vi "Traverse QSM - Nano.vi"(8 "error in":errorcluster, 10 "Nachrichten-Queues (Eingang)":T1) -> (0 "error out":errorcluster)   [LabVIEW 2014]
uses:
  All Message Queues.ctl
  Documents/LabVIEW Data/Unbenanntes Projekt 8/support/Message Queue/Message Cluster.ctl
  Documents/LabVIEW Data/Unbenanntes Projekt 8/support/Message Queue/Enqueue Message (Single).vi
  Documents/LabVIEW Data/Unbenanntes Projekt 8/support/Message Queue/Message Queue.lvlib
panel:
  out "i Blink":i32
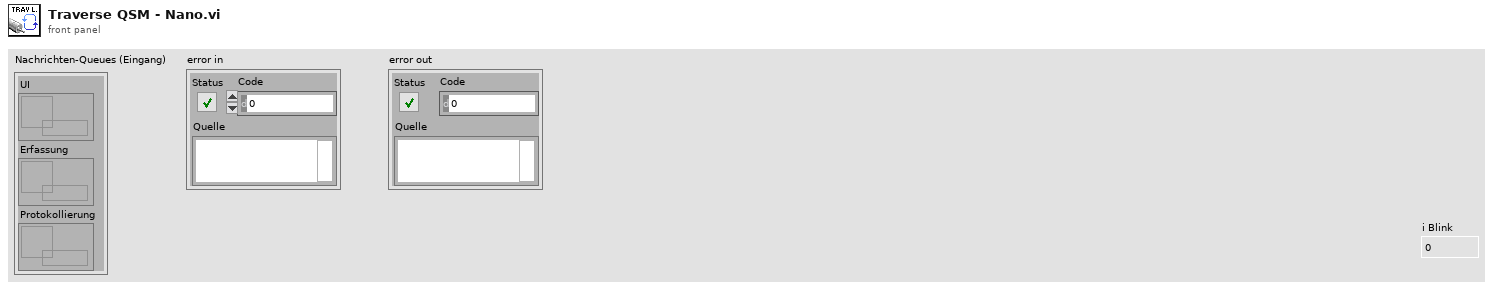
[diagram p1: front panel]
types:
  T1 = typedef "Message Queue.lvlib/All Message Queues.ctl" = cluster{"UI":refnum<queue>, "Erfassung":refnum<queue>, "Traverse":refnum<queue>}
  T2 = cluster{"Status":bool, "Code":i32, "Quelle":string}
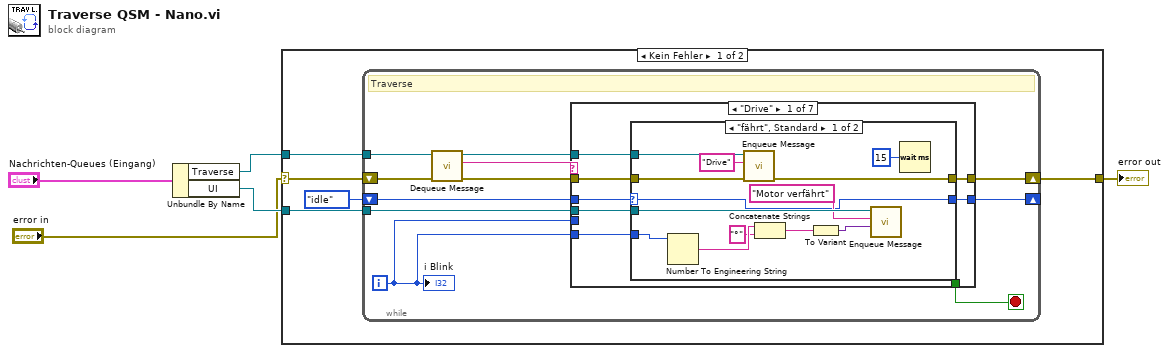
[diagram p0: block diagram]
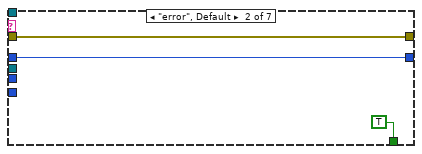
[diagram p3: hidden frame]
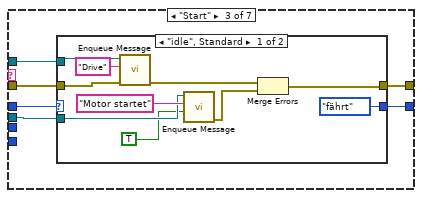
[diagram p4: hidden frame]
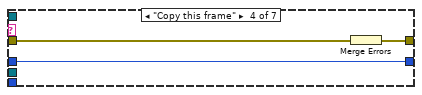
[diagram p6: hidden frame]
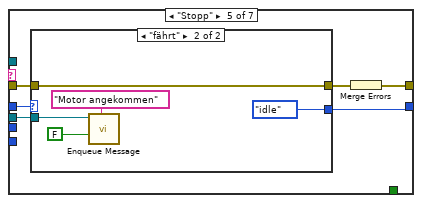
[diagram p7: hidden frame]
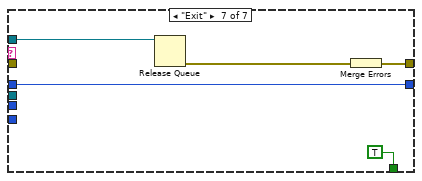
[diagram p10: hidden frame]
diagram:
  n1 = Unbundle By Name("Nachrichten-Queues (Eingang)") -> ("Traverse"=w4:refnum<queue>, "UI"=w3:refnum<queue>)
  n2 = case shown="Kein Fehler" "error in" {
    selector: "error in" -> [w6 w88]
    tunnel: w4 -> [w9 _]
    tunnel: w3 -> [w8 _]
    tunnel: [w7 w88] -> w2
    frame No Error {
      n3 = while {
        tunnel: w9 -> [w21]
        shift-right: [w17] -> w7
        shift-left: w6 -> [w16]
        shift-right: [w15] -> _
        shift-left: enum16{"idle", "fährt"}."idle" -> [w19]
        tunnel: w8 -> [w13]
        i -> [w12]
        stop <- w11 stop-if-true
        # "Traverse"
        n4 = call "Dequeue Message.vi"("error in (no error)"=w16, "Nachrichten-Queue"=w21) -> ("error out"=w18:T2, "Nachricht"=w20:string, "Nachrichten-Queue (Kopie)"=w14:refnum<queue>)  [unwired: 6 in, 1 out]
        n5 = case shown="\"Drive\"" w20 {
          tunnel: w12 -> [_ _ _ _ _ _ _]
          tunnel: w19 -> [w28 w45 w50 w65 w72 w81 w86]
          tunnel: w18 -> [w26 w46 w52 w67 w70 w82 _]
          tunnel: [w25 w46 w51 w66 w73 w82 w87] -> w17
          tunnel: [w27 w45 w49 w65 w71 w81 w86] -> w15
          tunnel: w14 -> [w24 _ w48 _ _ _ w85]
          tunnel: w13 -> [w23 _ w47 _ w68 _ _]
          tunnel: w12 -> [w22 _ _ _ _ _ _]
          tunnel: [_ TRUE _ _ _ _ TRUE] -> w11
          frame "Drive" {
            n6 = case shown="\"fährt\", Standard" w28 {
              selector: w28 -> [w33 w43]
              tunnel: [w33 w43] -> w27
              tunnel: w26 -> [w39 w42]
              tunnel: [w38 w42] -> w25
              tunnel: w24 -> [w40 _]
              tunnel: w23 -> [w37 _]
              tunnel: w22 -> [w31 _]
              frame "fährt", Default {
                n7 = Number To Engineering String(4:w31) -> (0:w30:string)  [unwired: 3 in]
                n8 = call-poly "Enqueue Message.vi"("error in (no error)"=w39, "Nachricht"="Drive", "Nachrichten-Queue"=w40) -> ("error out"=w38:T2)  [unwired: 7 in, 1 out]
                n9 = Concatenate Strings(w30, "°" ("String")) -> (w36:string)
                n10 = To Variant(anything=w36) -> (Variant=w35:variant)
                n11 = call-poly "Enqueue Message.vi"("Nachrichtendaten"=w35, "Nachricht"="Motor verfährt", "Nachrichten-Queue"=w37) -> ()  [unwired: 7 in, 2 out]
                n12 = Wait (ms)(milliseconds to wait=u32 15 ("Zu wartende ms")) -> ()  [unwired: 1 out]
              }
              frame "idle" {
              }
            }
          }
          frame "error", Default {
          }
          frame "Start" {
            n13 = case shown="\"idle\", Standard" w50 {
              selector: w50 -> [_ w63]
              tunnel: w52 -> [w60 w64]
              tunnel: [w58 w64] -> w51
              tunnel: [enum16{"idle", "fährt"}."fährt" w63] -> w49
              tunnel: w48 -> [w62 _]
              tunnel: w47 -> [w55 _]
              frame "idle", Default {
                n14 = call-poly "Enqueue Message.vi"("error in (no error)"=w60, "Nachricht"="Drive", "Nachrichten-Queue"=w62) -> ("error out"=w59:T2)  [unwired: 7 in, 1 out]
                n15 = call-poly "Enqueue Message.vi"("Nachrichtendaten"=TRUE ("Blinkend"), "Nachricht"="Motor startet", "Nachrichten-Queue"=w55) -> ("error out"=w53:T2)  [unwired: 7 in, 1 out]
                n16 = Merge Errors(w59, w53) -> (w58:errorcluster)
              }
              frame "fährt" {
              }
            }
          }
          frame "Copy this frame" {
            n17 = Merge Errors(w67) -> (w66:errorcluster)
          }
          frame "Stopp" {
            n18 = case shown="\"fährt\"" w72 {
              selector: w72 -> [w74 _]
              tunnel: [w74 enum16{"idle", "fährt"}."idle"] -> w71
              tunnel: w70 -> [w75 w79]
              tunnel: [w75 w79] -> w69
              tunnel: w68 -> [_ w78]
              frame "idle", Default {
              }
              frame "fährt" {
                n19 = call-poly "Enqueue Message.vi"("Nachrichtendaten"=FALSE ("Blinkend"), "Nachricht"="Motor angekommen", "Nachrichten-Queue"=w78) -> ()  [unwired: 7 in, 2 out]
              }
            }
            n20 = Merge Errors(w69) -> (w73:errorcluster)
          }
          frame "Initialize" {
          }
          frame "Exit" {
            n21 = Release Queue(queue=w85) -> (error out=w84:errorcluster)  [unwired: 2 in, 2 out]
            n22 = Merge Errors(w84) -> (w87:errorcluster)
          }
        }
        "i Blink" <- w12
      }
    }
    frame Error {
    }
  }
  "error out" <- w2
